vi "RFSA_Control.vi"(8 "error in (no error)":errorcluster, 10 "Device Resources":T1={"RFSG Resource in"="5646R", "RFSA Resource in"="5646R", "RFmx Resource in"=""}, 11 "Message_Queues":T2) -> (0 "error out":errorcluster)   [LabVIEW 2014]
uses:
  02_Controls/Message_Queues.ctl
  02_Controls/Message_Data_Ctl.ctl
  15_DataManagement/Device_Resources.ctl
  15_DataManagement/Config_RFSA_Vertical.ctl
  15_DataManagement/Config_RFSA_IQ_Acq.ctl
  15_DataManagement/Config_RFSA_Spectrum_Acq.ctl
  <instrlib>/niRFSA/niRFSA.llb/niRFSA Trigger Terminals.ctl
  <instrlib>/niRFSA/niRFSA.llb/niRFSA Trigger DigEdge - Edge Values.ctl
  <instrlib>/niRFSA/niRFSA.llb/niRFSA Configure Digital Edge Ref Trigger.vi
  <instrlib>/niRFSA/niRFSA.llb/niRFSA Fetch IQ (Complex Cluster 1Rec 1Chan).vi
  <instrlib>/niRFSA/niRFSA.llb/niRFSA Read IQ (Complex Cluster 1Rec 1Chan).vi
panel:
  out "RFSG_Msg":string
  out "Message":string
  out "RFSA Resource out":refnum<k15>
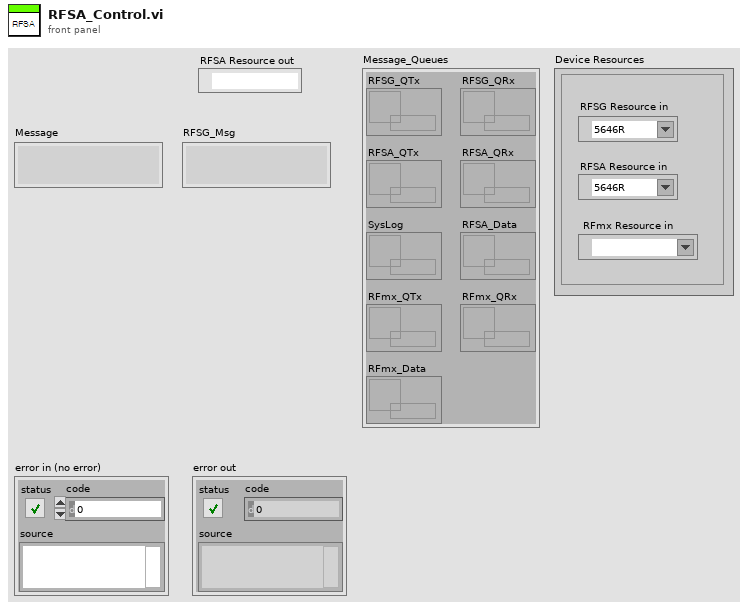
[diagram p1: front panel]
types:
  T1 = typedef "Device_Resources.ctl" = cluster{"RFSG Resource in":refnum<k15>, "RFSA Resource in":refnum<k15>, "RFmx Resource in":refnum<k15>}
  T2 = typedef "Message_Queues.ctl" = cluster{"RFSG_QTx":refnum<queue>, "RFSG_QRx":refnum<queue>, "RFSA_QTx":refnum<queue>, "RFSA_QRx":refnum<queue>, "SysLog":refnum<queue>, "RFSA_Data":refnum<queue>, "RFmx_QTx":refnum<queue>, "RFmx_QRx":refnum<queue>, "RFmx_Data":refnum<queue>}
  T3 = typedef "Config_RFSA_Vertical.ctl" = cluster{"Acquisition Type":i32, "Reference Level (dBm)":dbl, "External Gain (dB)":dbl}
  T4 = typedef "Config_RFSA_IQ_Acq.ctl" = cluster{"carrier frequency":dbl, "IQ rate (S/s)":dbl, "samples per record":i64}
  T5 = typedef "Config_RFSA_Spectrum_Acq.ctl" = cluster{"Resolution Bandwidth (Hz)":dbl, "Start Frequency (Hz)":dbl, "Stop Frequency (Hz)":dbl}
  T6 = typedef "niRFSA Trigger Terminals.ctl" = string
  T7 = typedef "niRFSA Trigger DigEdge - Edge Values.ctl" = i32
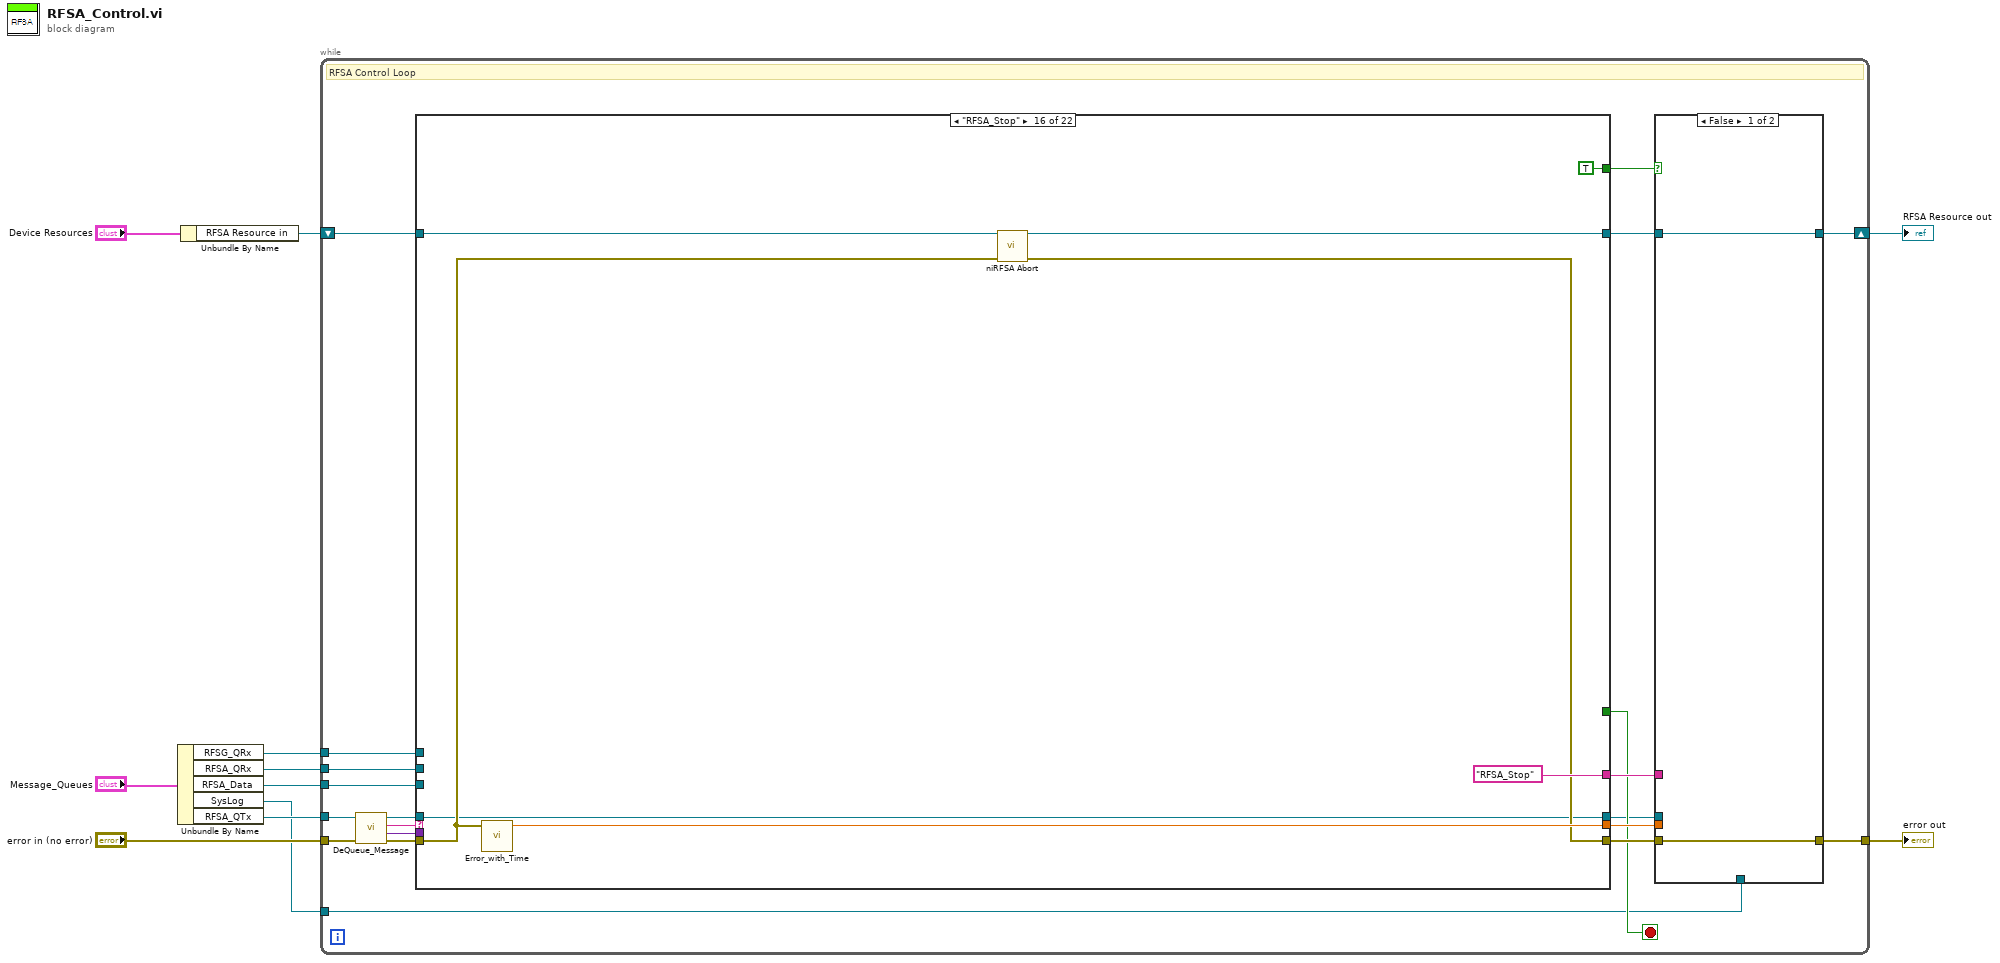
[diagram p0: block diagram]
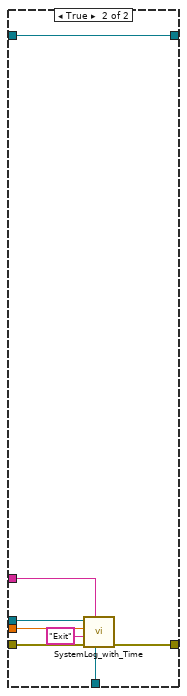
[diagram p2: hidden frame]
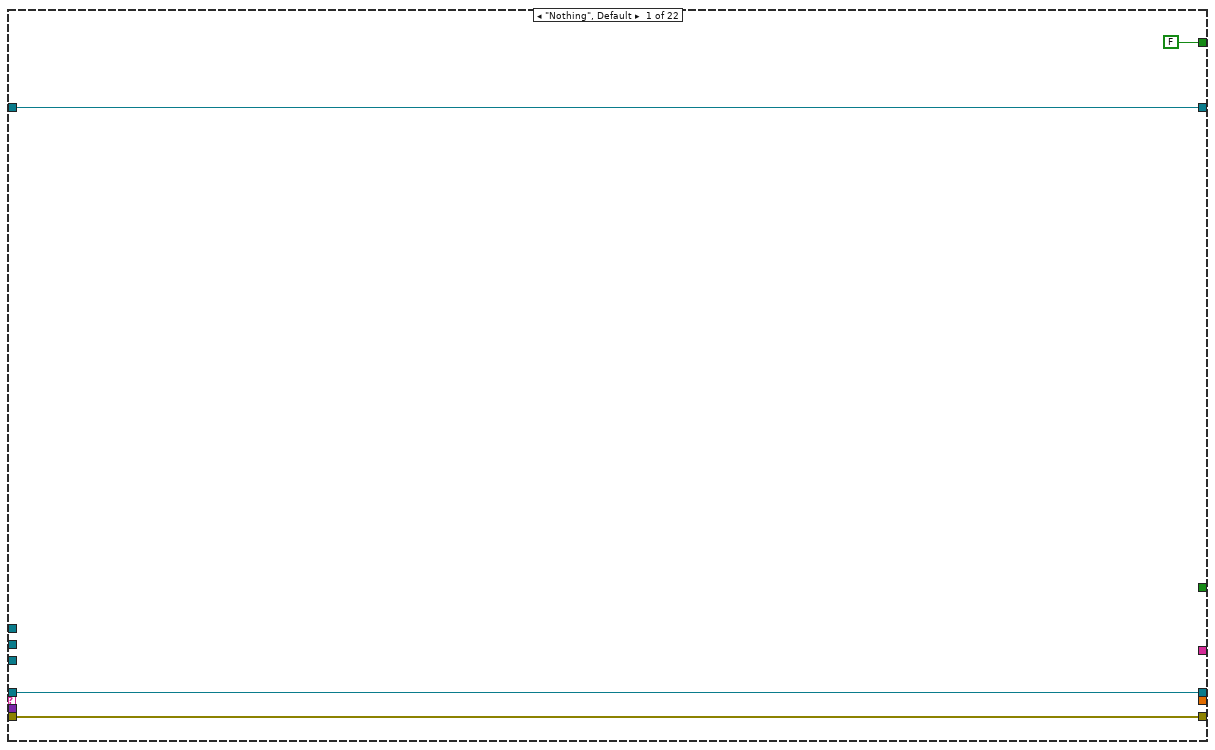
[diagram p3: hidden frame]
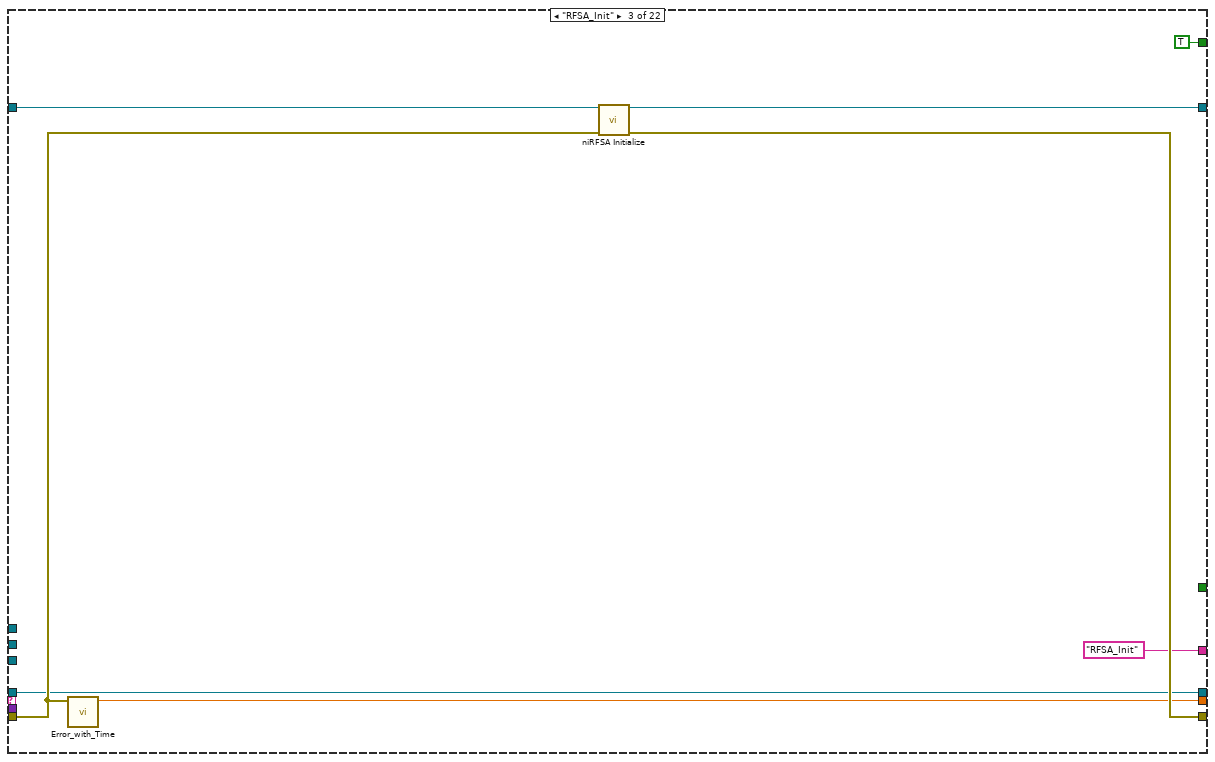
[diagram p5: hidden frame]
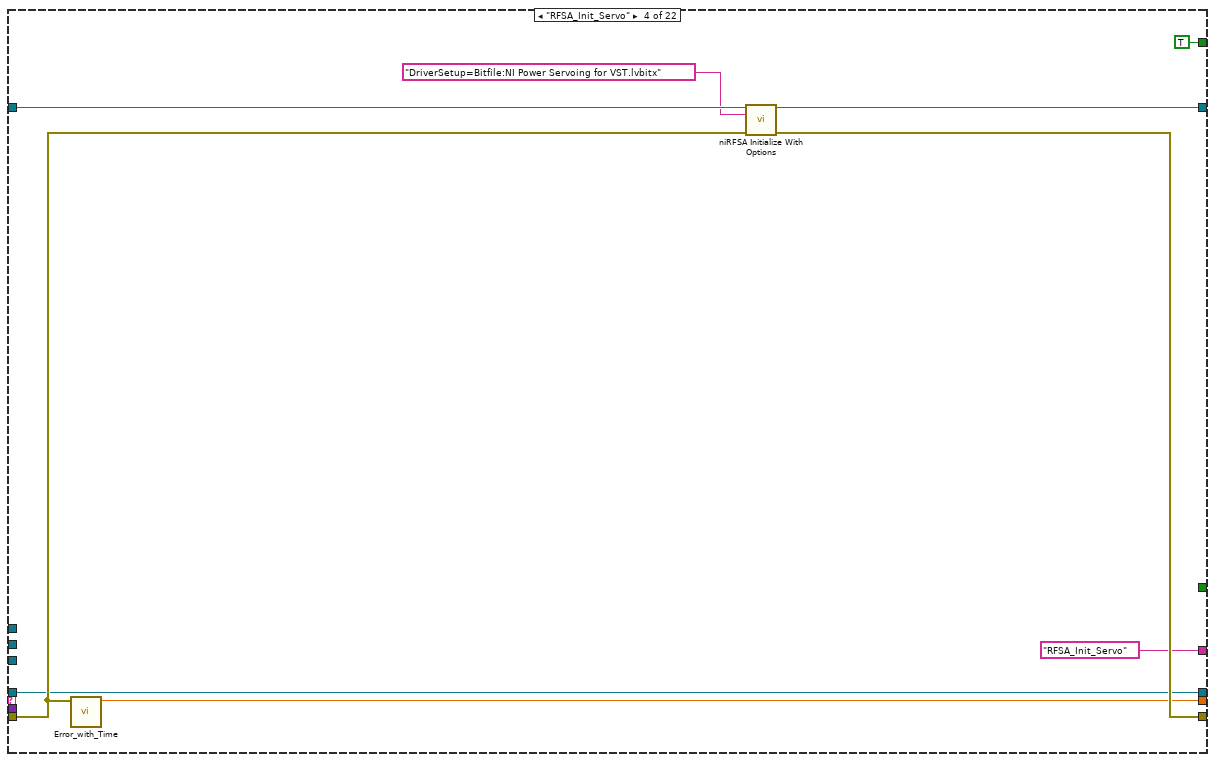
[diagram p6: hidden frame]
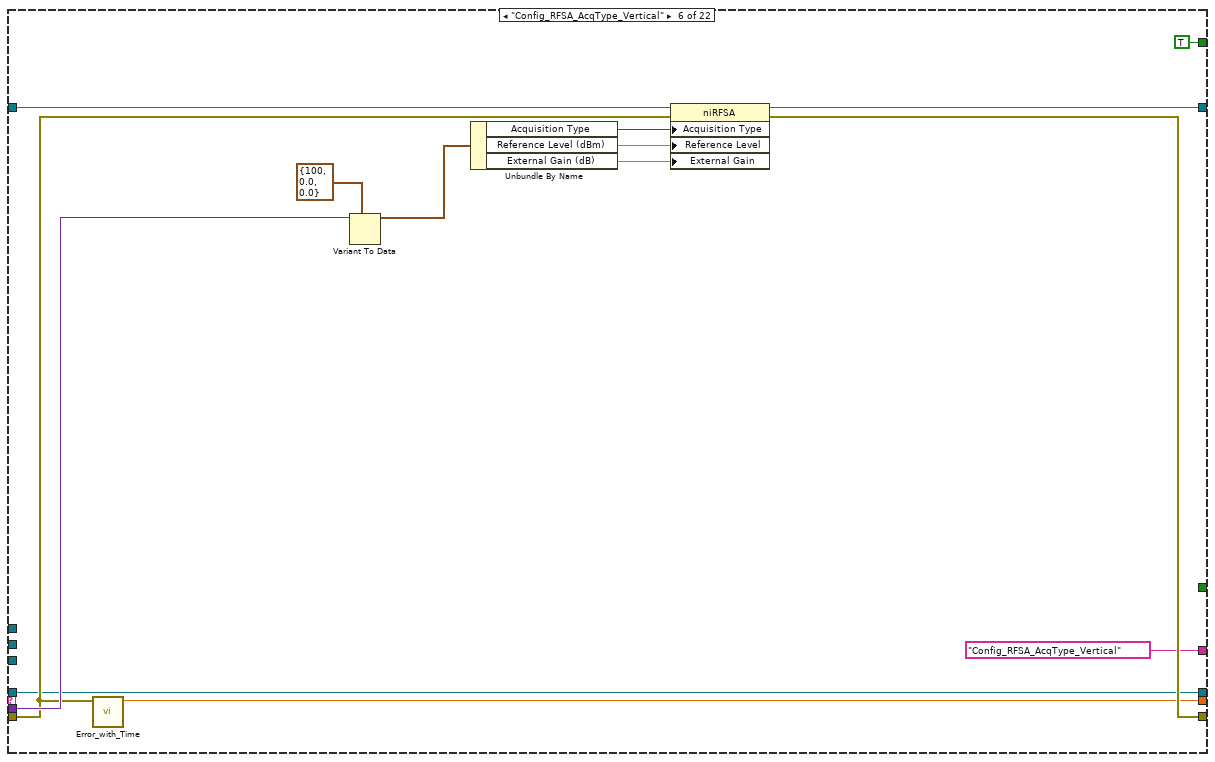
[diagram p8: hidden frame]
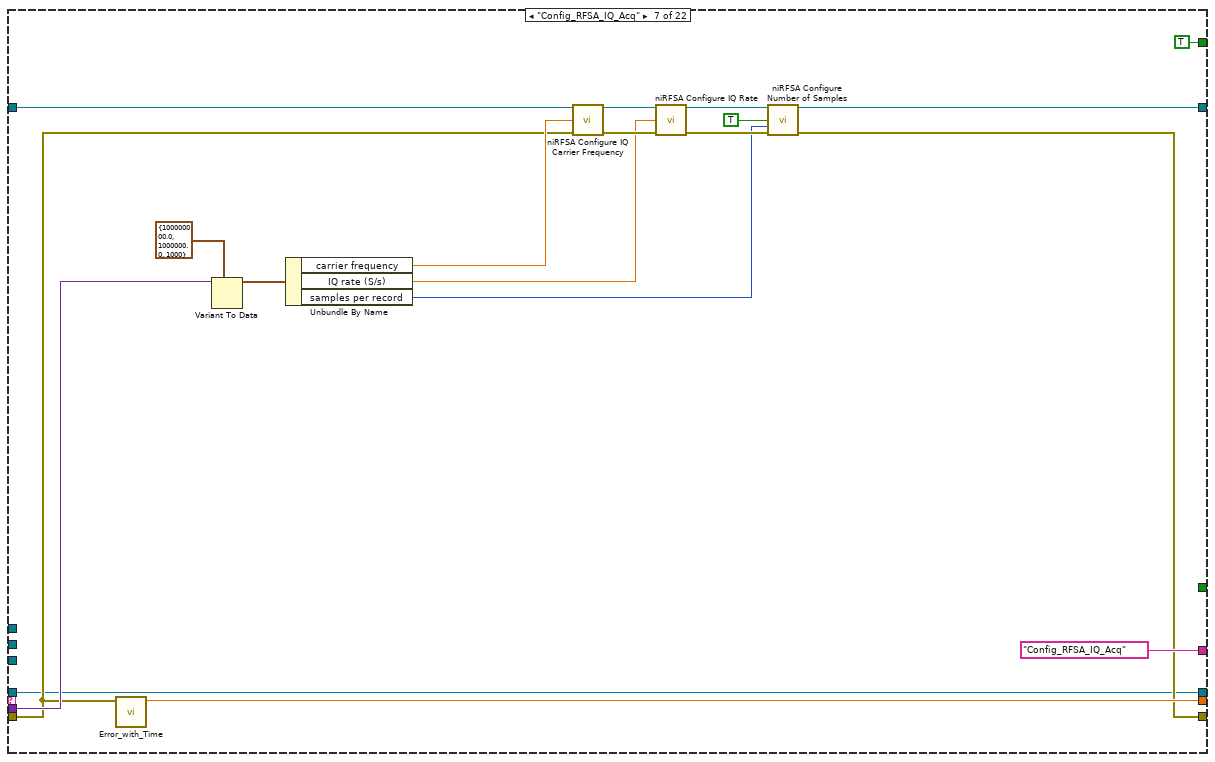
[diagram p9: hidden frame]
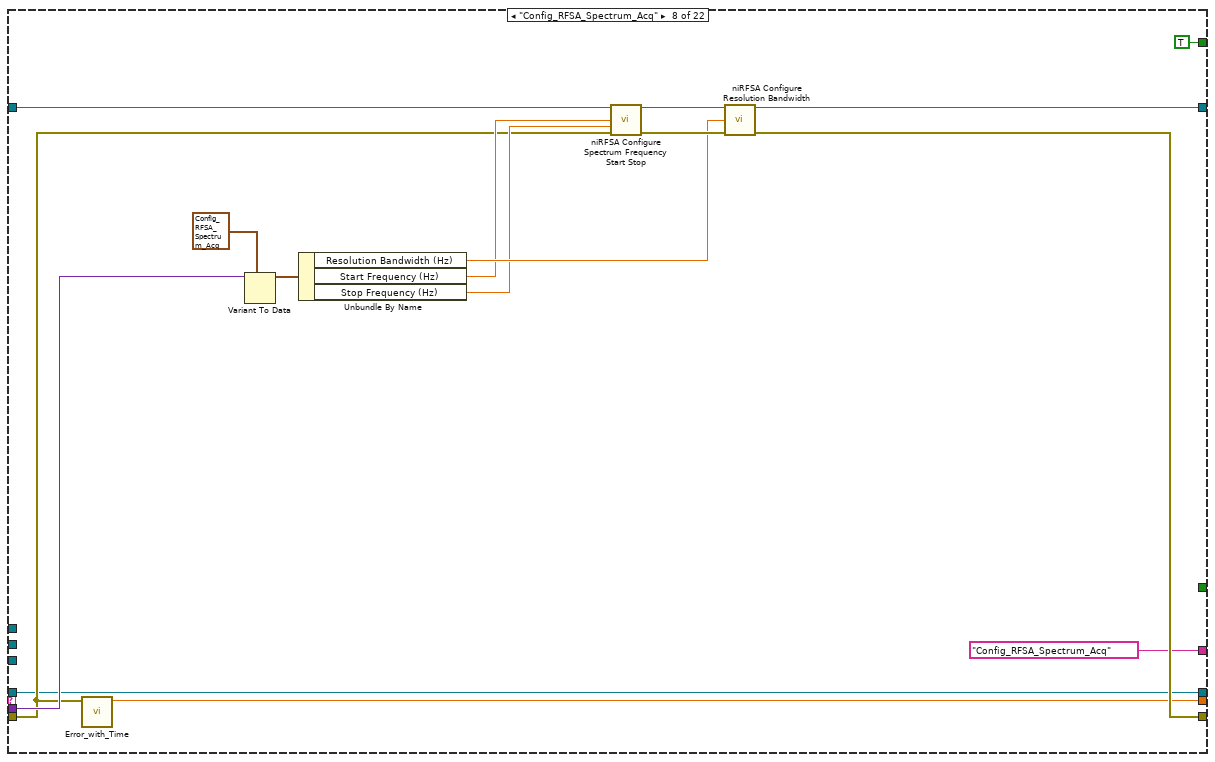
[diagram p10: hidden frame]
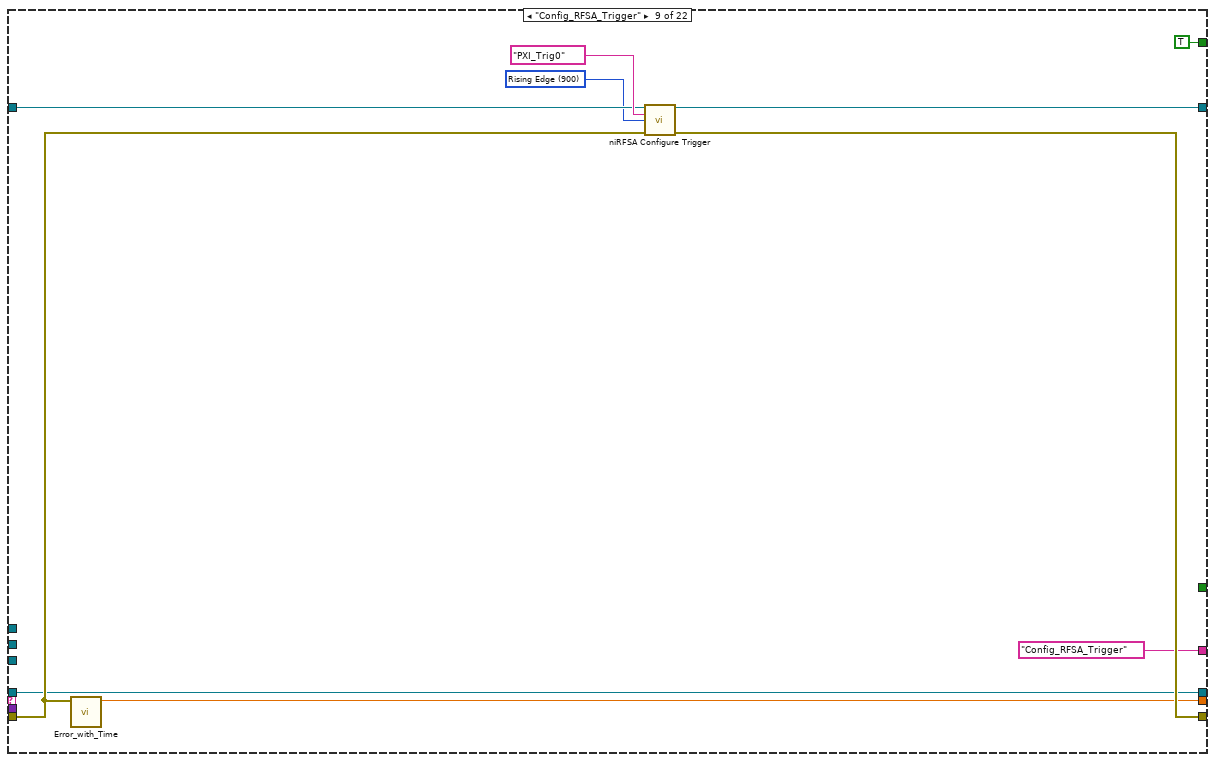
[diagram p11: hidden frame]
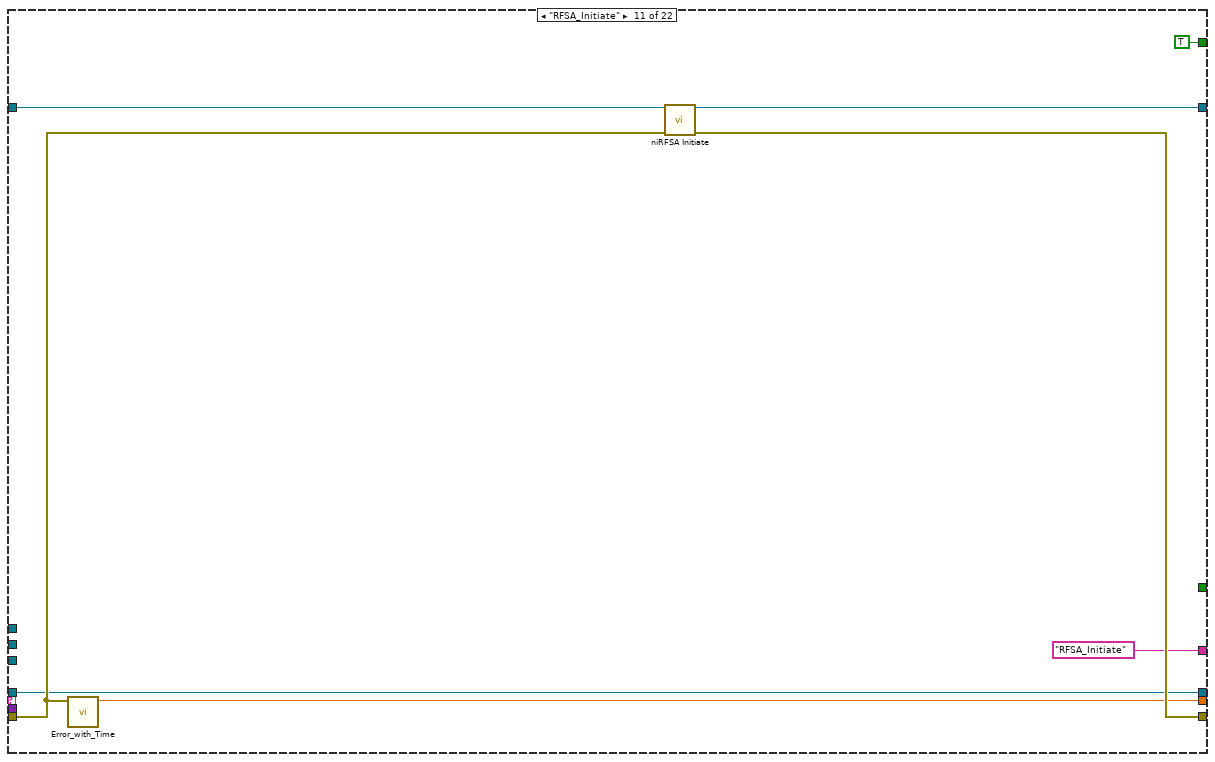
[diagram p13: hidden frame]
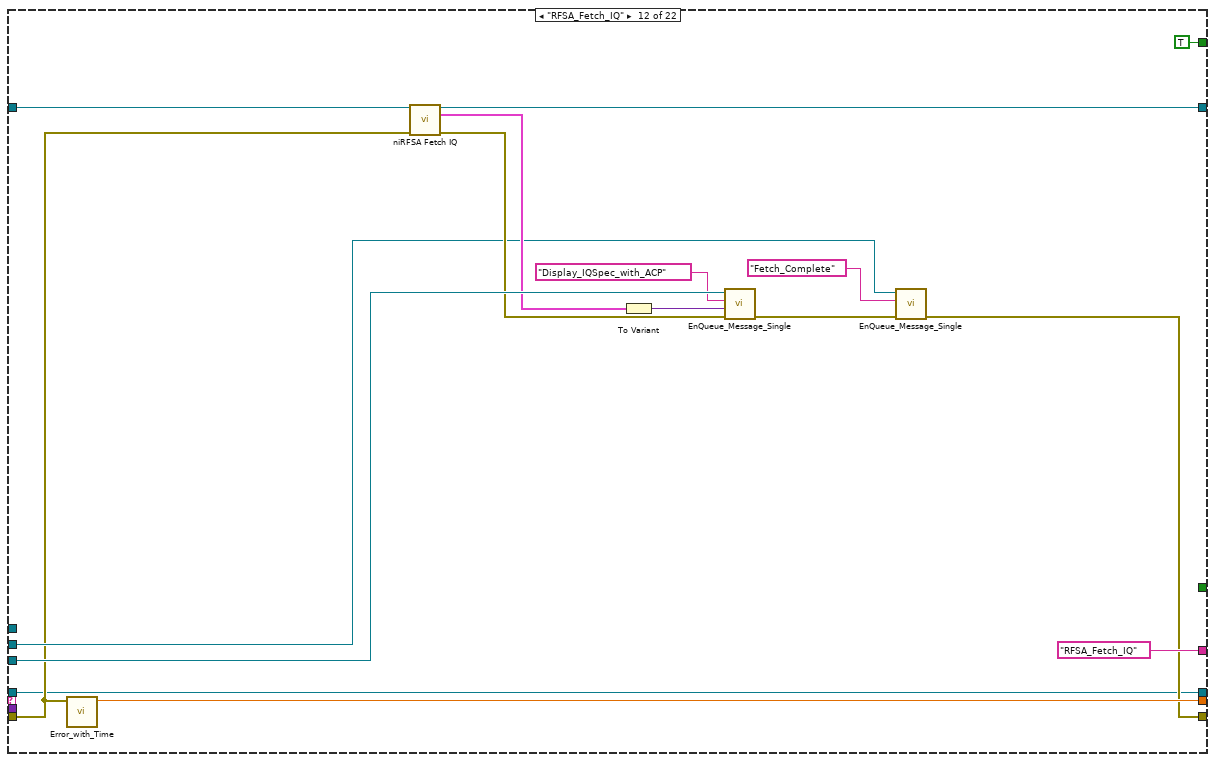
[diagram p14: hidden frame]
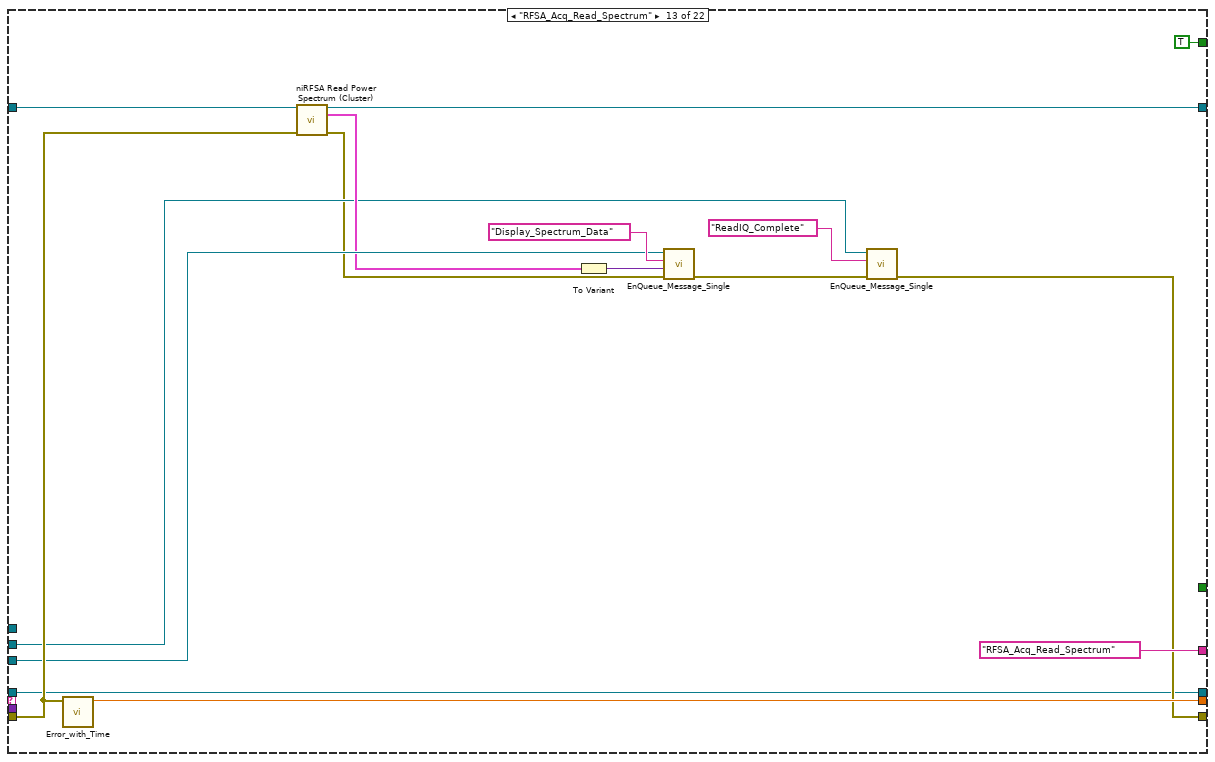
[diagram p15: hidden frame]
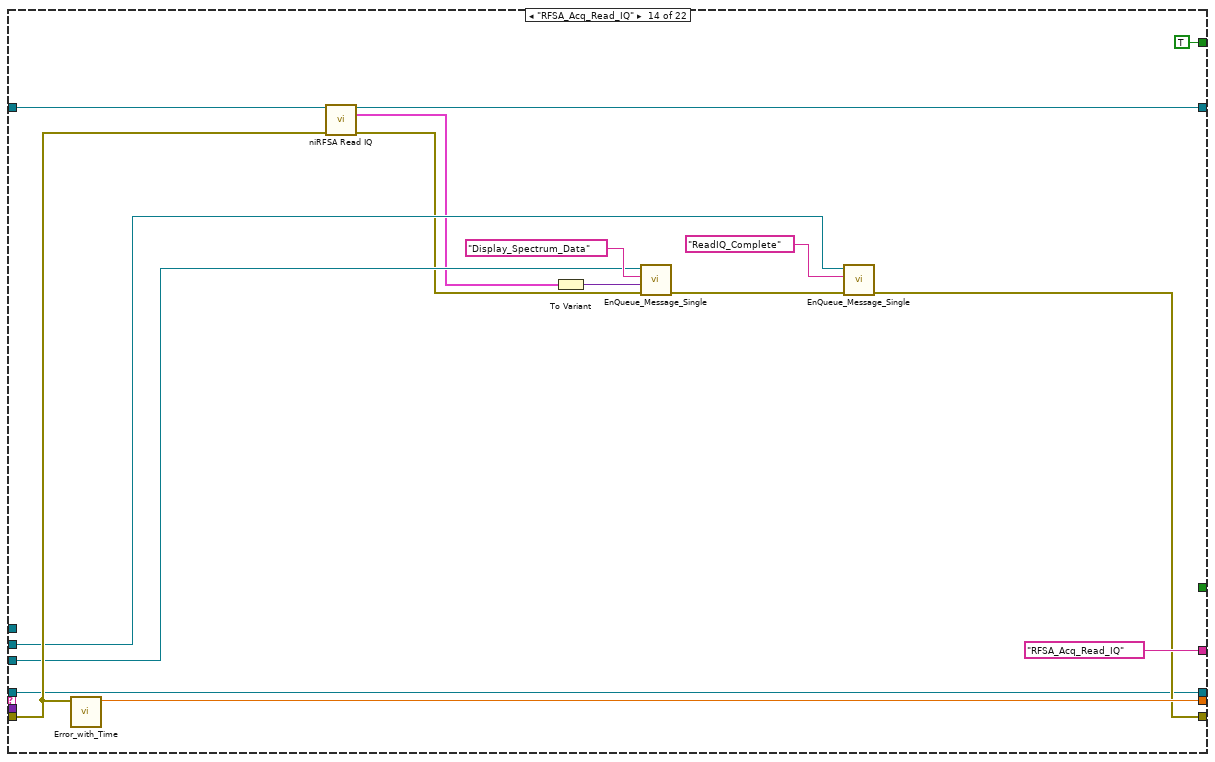
[diagram p16: hidden frame]
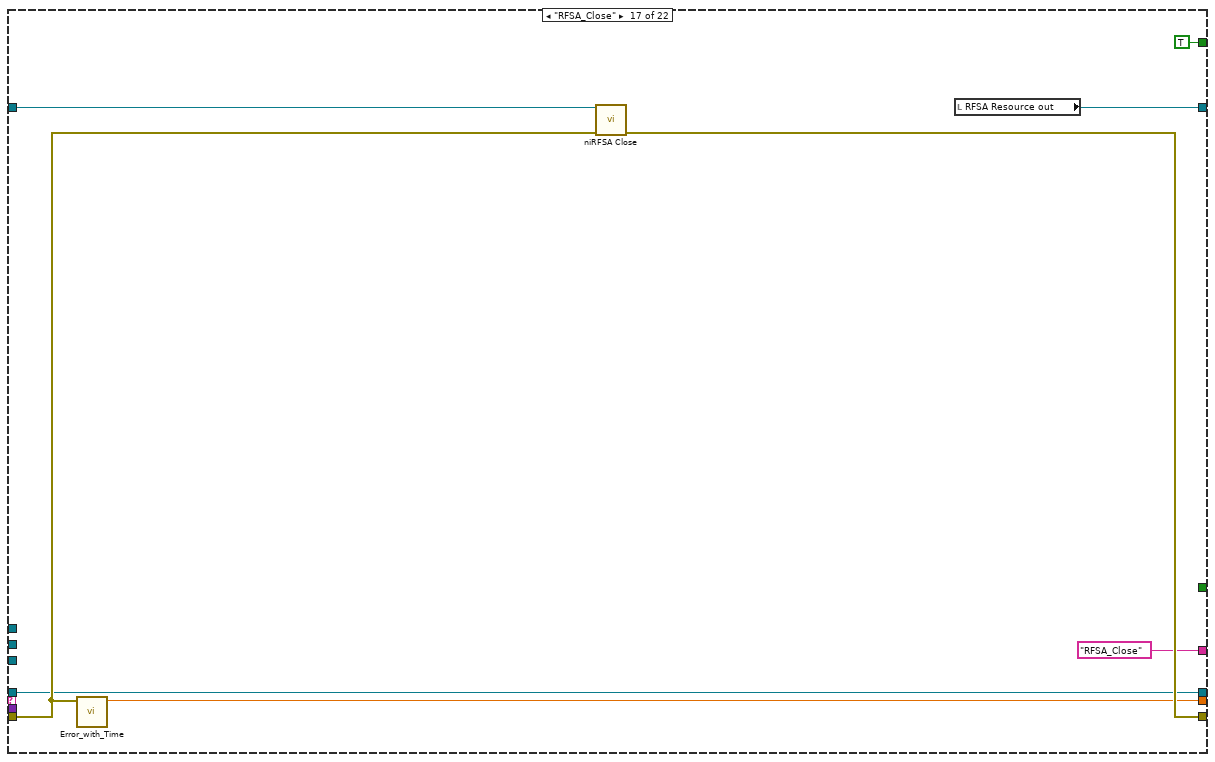
[diagram p18: hidden frame]
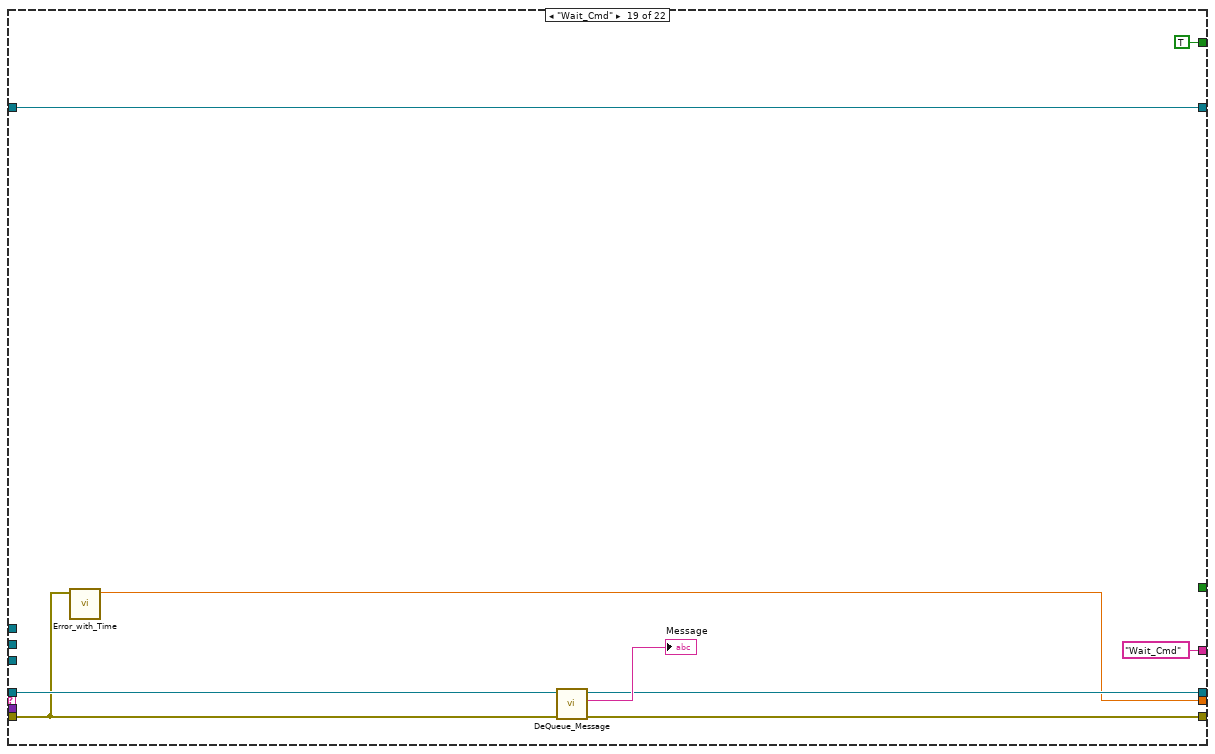
[diagram p20: hidden frame]
diagram:
  n1 = Unbundle By Name("Message_Queues") -> ("RFSG_QRx"=w3:refnum<queue>, "RFSA_QRx"=w5:refnum<queue>, "RFSA_Data"=w6:refnum<queue>, "SysLog"=w4:refnum<queue>, "RFSA_QTx"=w9:refnum<queue>)
  n2 = Unbundle By Name("Device Resources") -> ("RFSA Resource in"=w1:refnum<k15>)
  n3 = while {
    tunnel: "error in (no error)" -> [w31]
    tunnel: [w21] -> w10
    tunnel: w9 -> [w26]
    shift-right: [w12] -> w7
    shift-left: w1 -> [w25]
    tunnel: w6 -> [w24]
    tunnel: w5 -> [w23]
    tunnel: w4 -> [w16]
    tunnel: w3 -> [w18]
    stop <- w17 stop-if-true
    # "RFSA Control Loop"
    n4 = call "DeQueue_Message.vi"("error in (no error)"=w31, "Message_Queue"=w26) -> ("error out"=w27:errorcluster, "Message Data"=w29:variant, "Message"=w30:string, "Dup_Message_Queue"=w28:refnum<queue>)  [unwired: 6 in]
    n5 = case shown="\"RFSA_Stop\"" w30 {
      tunnel: w29 -> [_ _ _ _ _ w79 w95 w112 _ _ _ _ _ _ _ _ _ _ _ _ _ _]
      tunnel: w28 -> [w43 w46 w50 w58 w66 w70 w84 w103 w119 w128 w132 w140 w156 w172 w187 w191 w199 w206 w215 w222 w231 w238]
      tunnel: w27 -> [w45 w48 w51 w59 w67 w71 w88 w104 w120 w130 w133 w143 w166 w182 w188 w193 w200 w207 w210 w219 w228 w236]
      tunnel: [_ _ _ _ _ _ _ _ _ _ _ _ _ _ _ _ _ _ _ _ _ TRUE] -> w17
      tunnel: [w45 w48 w54 w63 w67 w80 w85 w107 w123 w130 w136 w141 w157 w173 w188 w192 w205 w207 w216 w225 w233 w236] -> w22
      tunnel: w25 -> [w44 w47 w56 w65 w68 w82 w96 w111 w126 w129 w138 w154 w170 w186 w189 w197 w204 w208 w217 w226 w235 w240]
      tunnel: [w44 w47 w55 w64 w68 w81 w86 w115 w124 w129 w137 w153 w169 w185 w189 w196 w202 w208 w217 w226 w235 w240] -> w13
      tunnel: w24 -> [_ _ _ _ _ _ _ _ _ _ _ w152 w161 w177 _ _ _ _ _ _ _ _]
      tunnel: w23 -> [_ _ _ _ _ _ _ _ _ _ _ w146 w159 w176 _ _ _ _ _ _ w232 _]
      tunnel: [_ _ "RFSA_Init" ("Message") "RFSA_Init_Servo" ("Message") _ "Config_RFSA_AcqType_Vertical" ("Message") "Config_RFSA_IQ_Acq" ("Message") "Config_RFSA_Spectrum_Acq" ("Message") "Config_RFSA_Trigger" ("Message") _ "RFSA_Initiate" ("Message") "RFSA_Fetch_IQ" ("Message") "RFSA_Acq_Read_Spectrum" ("Message") "RFSA_Acq_Read_IQ" ("Message") _ "RFSA_Stop" ("Message") "RFSA_Close" ("Message") _ "Wait_Cmd" ("Message") "Wait_RFSG" ("Message") "Send_to_Cmd" ("Message") "RFSA_Exit" ("Message")] -> w20
      tunnel: [_ _ w52 w60 _ w72 w89 w105 w121 _ w134 w144 w167 w183 _ w194 w201 _ w209 w218 w227 w237] -> w19
      tunnel: w18 -> [_ _ _ _ _ _ _ _ _ _ _ _ _ _ _ _ _ _ _ w223 _ _]
      tunnel: [w43 w46 w50 w58 w66 w70 w84 w103 w119 w128 w132 w140 w156 w172 w187 w191 w199 w206 w213 w222 w231 w238] -> w15
      tunnel: [FALSE _ TRUE TRUE _ TRUE TRUE TRUE TRUE _ TRUE TRUE TRUE TRUE _ TRUE TRUE _ TRUE TRUE TRUE _] -> w14
      frame "Nothing", Default {
      }
      frame "===== Device Init =====" {
      }
      frame "RFSA_Init" {
        n6 = call "Error_with_Time.vi"("error in (no error)"=w51) -> ("relative seconds"=w52:dbl)  [unwired: 10 in]
        n7 = call <instrlib>:"niRFSA Initialize.vi"("resource name"=w56, "error in"=w51) -> ("instrument handle"=w55:refnum<k15>, "error out"=w54:errorcluster)  [unwired: 12 in]
      }
      frame "RFSA_Init_Servo" {
        n8 = call "Error_with_Time.vi"("error in (no error)"=w59) -> ("relative seconds"=w60:dbl)  [unwired: 10 in]
        n9 = call <instrlib>:"niRFSA Initialize With Options.vi"("resource name"=w65, "option string"="DriverSetup=Bitfile:NI Power Servoing for VST.lvbitx" ("Bitfile"), "error in"=w59) -> ("instrument handle"=w64:refnum<k15>, "error out"=w63:errorcluster)  [unwired: 11 in]
      }
      frame "===== Configure =====" {
      }
      frame "Config_RFSA_AcqType_Vertical" {
        n10 = call "Error_with_Time.vi"("error in (no error)"=w71) -> ("relative seconds"=w72:dbl)  [unwired: 10 in]
        n11 = Variant To Data(type=T3 {"Acquisition Type"=100, "Reference Level (dBm)"=0.0, "External Gain (dB)"=0.0} ("Config_RFSA_Vertical"), Variant=w79) -> (data=w78:T3)  [unwired: 1 in, 1 out]
        n12 = Unbundle By Name(w78) -> ("Acquisition Type"=w77:i32, "Reference Level (dBm)"=w76:dbl, "External Gain (dB)"=w75:dbl)
        n13 = property class="niRFSA"(reference=w82, error in=w71, "Acquisition Type"=w77, "Reference Level"=w76, "External Gain"=w75) -> (reference out=w81:refnum<k15>, error out=w80:errorcluster)
      }
      frame "Config_RFSA_IQ_Acq" {
        n14 = call "Error_with_Time.vi"("error in (no error)"=w88) -> ("relative seconds"=w89:dbl)  [unwired: 10 in]
        n15 = Variant To Data(type=T4 {"carrier frequency"=100000000.0, "IQ rate (S/s)"=1000000.0, "samples per record"=1000} ("Config_RFSA_IQ_Acq"), Variant=w95) -> (data=w94:T4)  [unwired: 1 in, 1 out]
        n16 = Unbundle By Name(w94) -> ("carrier frequency"=w93:dbl, "IQ rate (S/s)"=w92:dbl, "samples per record"=w87:i64)
        n17 = call <instrlib>:"niRFSA Configure IQ Carrier Frequency.vi"("instrument handle"=w96, "carrier frequency"=w93, "error in"=w88) -> ("instrument handle out"=w99:refnum<k15>, "error out"=w98:errorcluster)  [unwired: 11 in]
        n18 = call <instrlib>:"niRFSA Configure IQ Rate.vi"("instrument handle"=w99, "IQ rate (S/s)"=w92, "error in"=w98) -> ("instrument handle out"=w101:refnum<k15>, "error out"=w100:errorcluster)  [unwired: 11 in]
        n19 = call <instrlib>:"niRFSA Configure Number of Samples.vi"("instrument handle"=w101, "number of samples is finite"=TRUE, "samples per record"=w87, "error in"=w100) -> ("instrument handle out"=w86:refnum<k15>, "error out"=w85:errorcluster)  [unwired: 10 in]
      }
      frame "Config_RFSA_Spectrum_Acq" {
        n20 = call "Error_with_Time.vi"("error in (no error)"=w104) -> ("relative seconds"=w105:dbl)  [unwired: 10 in]
        n21 = Variant To Data(type=T5 {"Resolution Bandwidth (Hz)"=10000.0, "Start Frequency (Hz)"=90000000.0, "Stop Frequency (Hz)"=110000000.0} ("Config_RFSA_Spectrum_Acq"), Variant=w112) -> (data=w114:T5)  [unwired: 1 in, 1 out]
        n22 = Unbundle By Name(w114) -> ("Resolution Bandwidth (Hz)"=w110:dbl, "Start Frequency (Hz)"=w109:dbl, "Stop Frequency (Hz)"=w108:dbl)
        n23 = call <instrlib>:"niRFSA Configure Spectrum Frequency Start Stop.vi"("instrument handle"=w111, "start frequency"=w109, "stop frequency"=w108, "error in"=w104) -> ("instrument handle out"=w117:refnum<k15>, "error out"=w116:errorcluster)  [unwired: 10 in]
        n24 = call <instrlib>:"niRFSA Configure Resolution Bandwidth.vi"("instrument handle"=w117, "resolution bandwidth (Hz)"=w110, "error in"=w116) -> ("instrument handle out"=w115:refnum<k15>, "error out"=w107:errorcluster)  [unwired: 11 in]
      }
      frame "Config_RFSA_Trigger" {
        w125 = T7 900 items=["Rising Edge"=900, "Falling Edge"=901] ("edge")
        n25 = call "Error_with_Time.vi"("error in (no error)"=w120) -> ("relative seconds"=w121:dbl)  [unwired: 10 in]
        n26 = call-poly <instrlib>:"niRFSA Configure Trigger.vi"("instrument handle"=w126, "source"=T6 "PXI_Trig0", "edge"=w125, "error in"=w120) -> ("instrument handle out"=w124:refnum<k15>, "error out"=w123:errorcluster)  [unwired: 2 in, 8 out]
      }
      frame "===== Acquisition =====" {
      }
      frame "RFSA_Initiate" {
        n27 = call "Error_with_Time.vi"("error in (no error)"=w133) -> ("relative seconds"=w134:dbl)  [unwired: 10 in]
        n28 = call <instrlib>:"niRFSA Initiate.vi"("instrument handle"=w138, "error in"=w133) -> ("instrument handle out"=w137:refnum<k15>, "error out"=w136:errorcluster)  [unwired: 12 in]
      }
      frame "RFSA_Fetch_IQ" {
        n29 = call "Error_with_Time.vi"("error in (no error)"=w143) -> ("relative seconds"=w144:dbl)  [unwired: 10 in]
        n30 = call-poly <instrlib>:"niRFSA Fetch IQ.vi"("instrument handle"=w154, "error in"=w143) -> ("instrument handle out"=w153:refnum<k15>, "data"=w148:cluster{"t0":dbl, "dt":dbl, "Y":cdb[]}, "error out"=w149:errorcluster)  [unwired: 3 in, 8 out]
        n31 = To Variant(anything=w148) -> (Variant=w151:variant)
        n32 = call "EnQueue_Message_Single.vi"("error in (no error)"=w149, "Message Data"=w151, "Message"="Display_IQSpec_with_ACP", "Message_Queue"=w152) -> ("error out"=w142:errorcluster)  [unwired: 6 in, 1 out]
        n33 = call "EnQueue_Message_Single.vi"("error in (no error)"=w142, "Message"="Fetch_Complete", "Message_Queue"=w146) -> ("error out"=w141:errorcluster)  [unwired: 7 in, 1 out]
      }
      frame "RFSA_Acq_Read_Spectrum" {
        n34 = call "Error_with_Time.vi"("error in (no error)"=w166) -> ("relative seconds"=w167:dbl)  [unwired: 10 in]
        n35 = call <instrlib>:"niRFSA Read Power Spectrum (Cluster).vi"("instrument handle"=w170, "error in"=w166) -> ("instrument handle out"=w169:refnum<k15>, "power spectrum"=w160:cluster{"f0":dbl, "df":dbl, "data":dbl[]}, "error out"=w158:errorcluster)  [unwired: 11 in]
        n36 = To Variant(anything=w160) -> (Variant=w165:variant)
        n37 = call "EnQueue_Message_Single.vi"("error in (no error)"=w158, "Message Data"=w165, "Message"="Display_Spectrum_Data", "Message_Queue"=w161) -> ("error out"=w162:errorcluster)  [unwired: 6 in, 1 out]
        n38 = call "EnQueue_Message_Single.vi"("error in (no error)"=w162, "Message"="ReadIQ_Complete", "Message_Queue"=w159) -> ("error out"=w157:errorcluster)  [unwired: 7 in, 1 out]
      }
      frame "RFSA_Acq_Read_IQ" {
        n39 = call "Error_with_Time.vi"("error in (no error)"=w182) -> ("relative seconds"=w183:dbl)  [unwired: 10 in]
        n40 = call-poly <instrlib>:"niRFSA Read IQ.vi"("instrument handle"=w186, "error in"=w182) -> ("instrument handle out"=w185:refnum<k15>, "data"=w175:cluster{"t0":dbl, "dt":dbl, "Y":cdb[]}, "error out"=w174:errorcluster)  [unwired: 11 in]
        n41 = To Variant(anything=w175) -> (Variant=w181:variant)
        n42 = call "EnQueue_Message_Single.vi"("error in (no error)"=w174, "Message Data"=w181, "Message"="Display_Spectrum_Data", "Message_Queue"=w177) -> ("error out"=w178:errorcluster)  [unwired: 6 in, 1 out]
        n43 = call "EnQueue_Message_Single.vi"("error in (no error)"=w178, "Message"="ReadIQ_Complete", "Message_Queue"=w176) -> ("error out"=w173:errorcluster)  [unwired: 7 in, 1 out]
      }
      frame "===== Sesion Stop&Close =====" {
      }
      frame "RFSA_Stop" {
        n44 = call "Error_with_Time.vi"("error in (no error)"=w193) -> ("relative seconds"=w194:dbl)  [unwired: 10 in]
        n45 = call <instrlib>:"niRFSA Abort.vi"("instrument handle"=w197, "error in"=w193) -> ("instrument handle out"=w196:refnum<k15>, "error out"=w192:errorcluster)  [unwired: 12 in]
      }
      frame "RFSA_Close" {
        n46 = call "Error_with_Time.vi"("error in (no error)"=w200) -> ("relative seconds"=w201:dbl)  [unwired: 10 in]
        n47 = call <instrlib>:"niRFSA Close.vi"("instrument handle"=w204, "error in"=w200) -> ("error out"=w205:errorcluster)  [unwired: 13 in]
        n48 = local read "RFSA Resource out"() -> (w202:refnum<k15>)
      }
      frame "===== Operation =====" {
      }
      frame "Wait_Cmd" {
        n49 = call "Error_with_Time.vi"("error in (no error)"=w210) -> ("relative seconds"=w209:dbl)  [unwired: 10 in]
        n50 = call "DeQueue_Message.vi"("error in (no error)"=w210, "Message_Queue"=w215) -> ("error out"=w216:errorcluster, "Message"=→"Message":string, "Dup_Message_Queue"=w213:refnum<queue>)  [unwired: 6 in, 1 out]
      }
      frame "Wait_RFSG" {
        n51 = call "Error_with_Time.vi"("error in (no error)"=w219) -> ("relative seconds"=w218:dbl)  [unwired: 10 in]
        n52 = call "DeQueue_Message.vi"("error in (no error)"=w219, "Message_Queue"=w223) -> ("error out"=w225:errorcluster, "Message"=→"RFSG_Msg":string)  [unwired: 6 in, 2 out]
      }
      frame "Send_to_Cmd" {
        n53 = call "Error_with_Time.vi"("error in (no error)"=w228) -> ("relative seconds"=w227:dbl)  [unwired: 10 in]
        n54 = call "EnQueue_Message_Single.vi"("error in (no error)"=w228, "Message"="OK", "Message_Queue"=w232) -> ("error out"=w233:errorcluster)  [unwired: 7 in, 1 out]
      }
      frame "Exit" {
        n55 = call "Error_with_Time.vi"("error in (no error)"=w236) -> ("relative seconds"=w237:dbl)  [unwired: 10 in]
      }
    }
    n56 = case shown="False" w14 {
      tunnel: w22 -> [w33 w41]
      tunnel: [w33 w40] -> w21
      tunnel: w20 -> [_ w39]
      tunnel: w15 -> [_ w38]
      tunnel: w19 -> [_ w37]
      tunnel: w16 -> [_ w36]
      tunnel: w13 -> [w32 w35]
      tunnel: [w32 w35] -> w12
      frame False {
      }
      frame True {
        n57 = call "SystemLog_with_Time.vi"("SysLog_Queue"=w36, "Message_in"=w39, "error in (no error)"=w41, "Send_Msg"="Exit", "Tick_in"=w37, "Worker_Queue"=w38) -> ("error out"=w40:errorcluster)  [unwired: 5 in]
      }
    }
  }
  "error out" <- w10
  "RFSA Resource out" <- w7
